vi "WFT Open.vi"(8 "Error In":errorcluster, 10 "idxDevice":i32) -> (0 "Error Out":errorcluster, 2 "ret":i32, 3 "WaveForms Session Out":T1)   [LabVIEW 2020, in "lv_waveforms_toolkit.lvlib"]
uses:
  lv_waveforms_toolkit.lvlib
  WFT Session.ctl
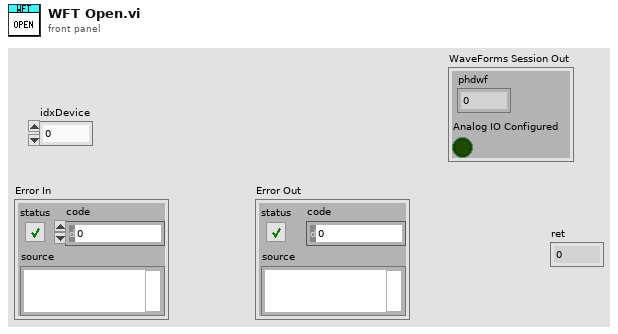
[diagram p1: front panel]
types:
  T1 = typedef "lv_waveforms_toolkit.lvlib/WFT Session.ctl" = cluster{"phdwf":i32, "Analog IO Configured":bool}
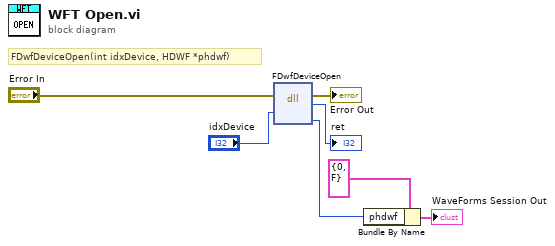
[diagram p0: block diagram]
diagram:
  # "FDwfDeviceOpen(int idxDevice, HDWF *phdwf)"
  n1 = dll-call lib="dwf" fn="FDwfDeviceOpen"(error in="Error In", "idxDevice"="idxDevice") -> (error out=→"Error Out":errorcluster, "return type"=→"ret":i32, "phdwf"=w1:i32)  [unwired: 4 in, 1 out]
  n2 = Bundle By Name(cluster=T1 {"phdwf"=0, "Analog IO Configured"=FALSE} ("WaveForms Session"), "phdwf"=w1) -> (→"WaveForms Session Out":T1)
